vi "柱塞泵调试界面.vi"() -> ()   [LabVIEW 2016, in "质控单元.lvlib"]
uses:
  <vilib>/Utility/miscctls.llb/LVPointTypeDef.ctl
  <vilib>/Analysis/6fits.llb/Curve Fitting Criteria.ctl
  <vilib>/Analysis/NI_AALPro.lvlib
panel:
  out "柱塞泵5体积":dbl
  out "柱塞泵4体积":dbl
  out "柱塞泵3体积":dbl
  out "柱塞泵2体积":dbl
  out "柱塞泵1体积":dbl
  in  "B 5":dbl caption="B5"
  in  "K 5":dbl caption="K5"
  in  "柱塞泵5":bool
  out "关闭 2":bool=TRUE
  in  "枚举":enum16{"柱塞泵1", "柱塞泵2", "柱塞泵3", "柱塞泵4"}(ring)
  in  "柱塞泵4":bool
  in  "柱塞泵3":bool
  in  "柱塞泵2":bool
  in  "柱塞泵1":bool
  out "线性值":T1
  in  "读取":bool
  in  "写入":bool
  in  "柱塞泵枚举":enum16{"柱塞泵1", "柱塞泵2", "柱塞泵3", "柱塞泵4", "柱塞泵5"}(ring)
  in  "启用计算":bool
  in  "标准体积 2":dbl
  in  "标准体积 3":dbl
  in  "实际体积 1":dbl
  in  "实际体积 2":dbl
  in  "实际体积 3":dbl
  in  "标准体积 4":dbl
  in  "实际体积 4":dbl
  in  "标准体积 5":dbl
  in  "实际体积 5":dbl
  in  "标准体积 1":dbl
  out "拟合方程":string
  out "r^2":dbl format="%_6g"
  in  "B 4":dbl caption="B4"
  in  "K 4":dbl caption="K4"
  in  "B 3":dbl caption="B3"
  in  "K 3":dbl caption="K3"
  in  "B 2":dbl caption="B2"
  in  "K 2":dbl caption="K2"
  in  "B":dbl caption="B1"
  in  "K":dbl caption="K1"
  in  "关闭":bool
  # "柱塞泵手动调试计算界面"
  # "柱塞泵启动控制"
  # "柱塞泵体积："
  # "柱塞泵5点线性计算"
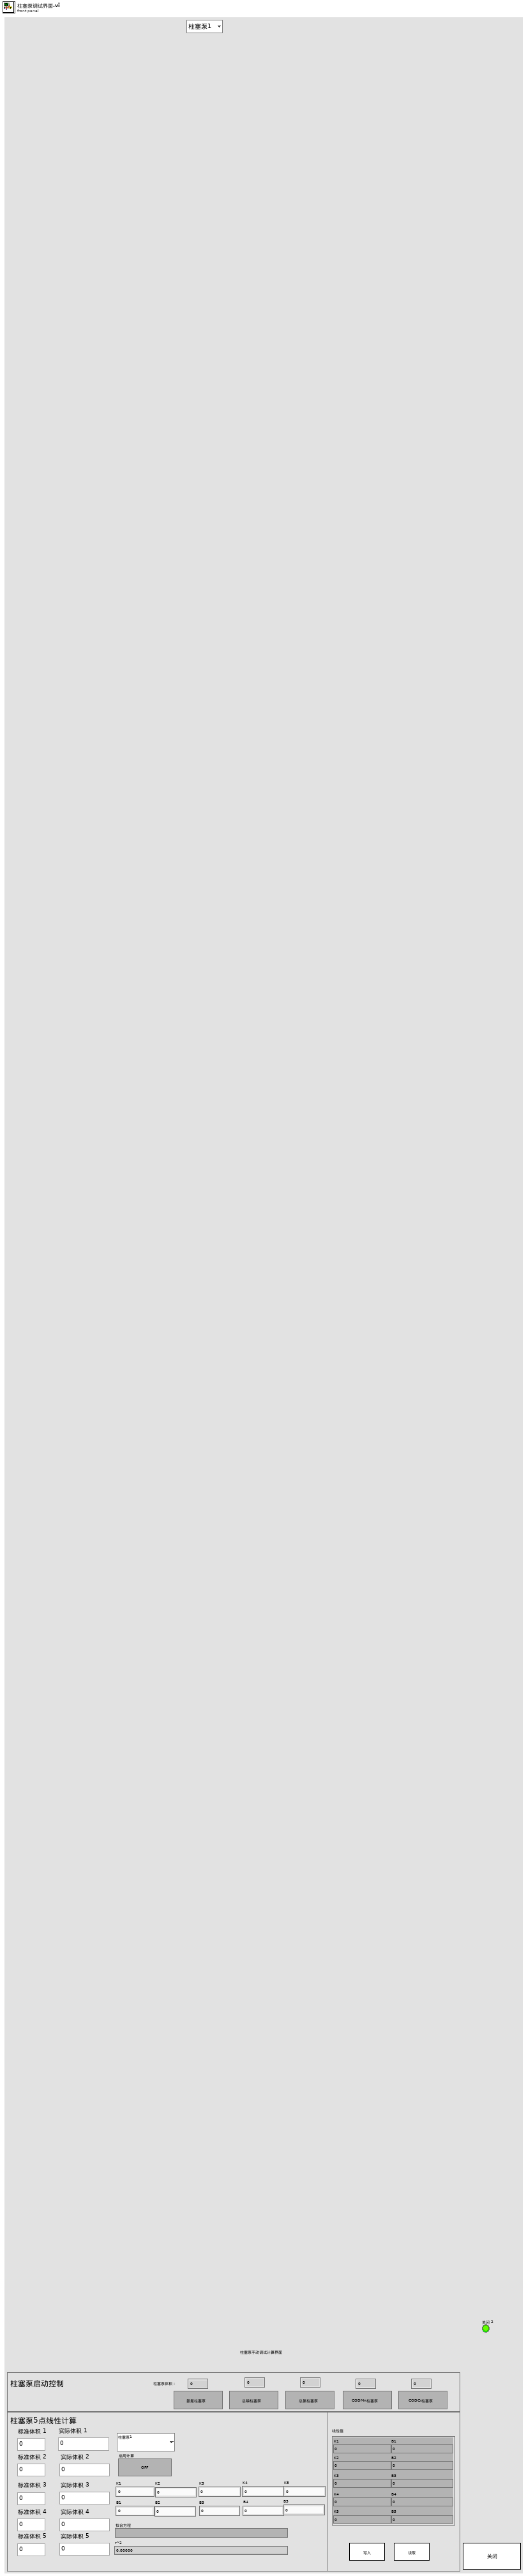
[diagram p1: front panel]
types:
  T1 = cluster{"K1":sgl, "B1":sgl, "K2":sgl, "B2":sgl, "K3":sgl, "B3":sgl, "K4":sgl, "B4":sgl, "K5":sgl, "B5":sgl}
  T2 = typedef "LVPointTypeDef.ctl" = cluster{"Horizontal":i16, "Vertical":i16}
  T3 = typedef "NI_AALPro.lvlib/Curve Fitting Criteria.ctl" = u16
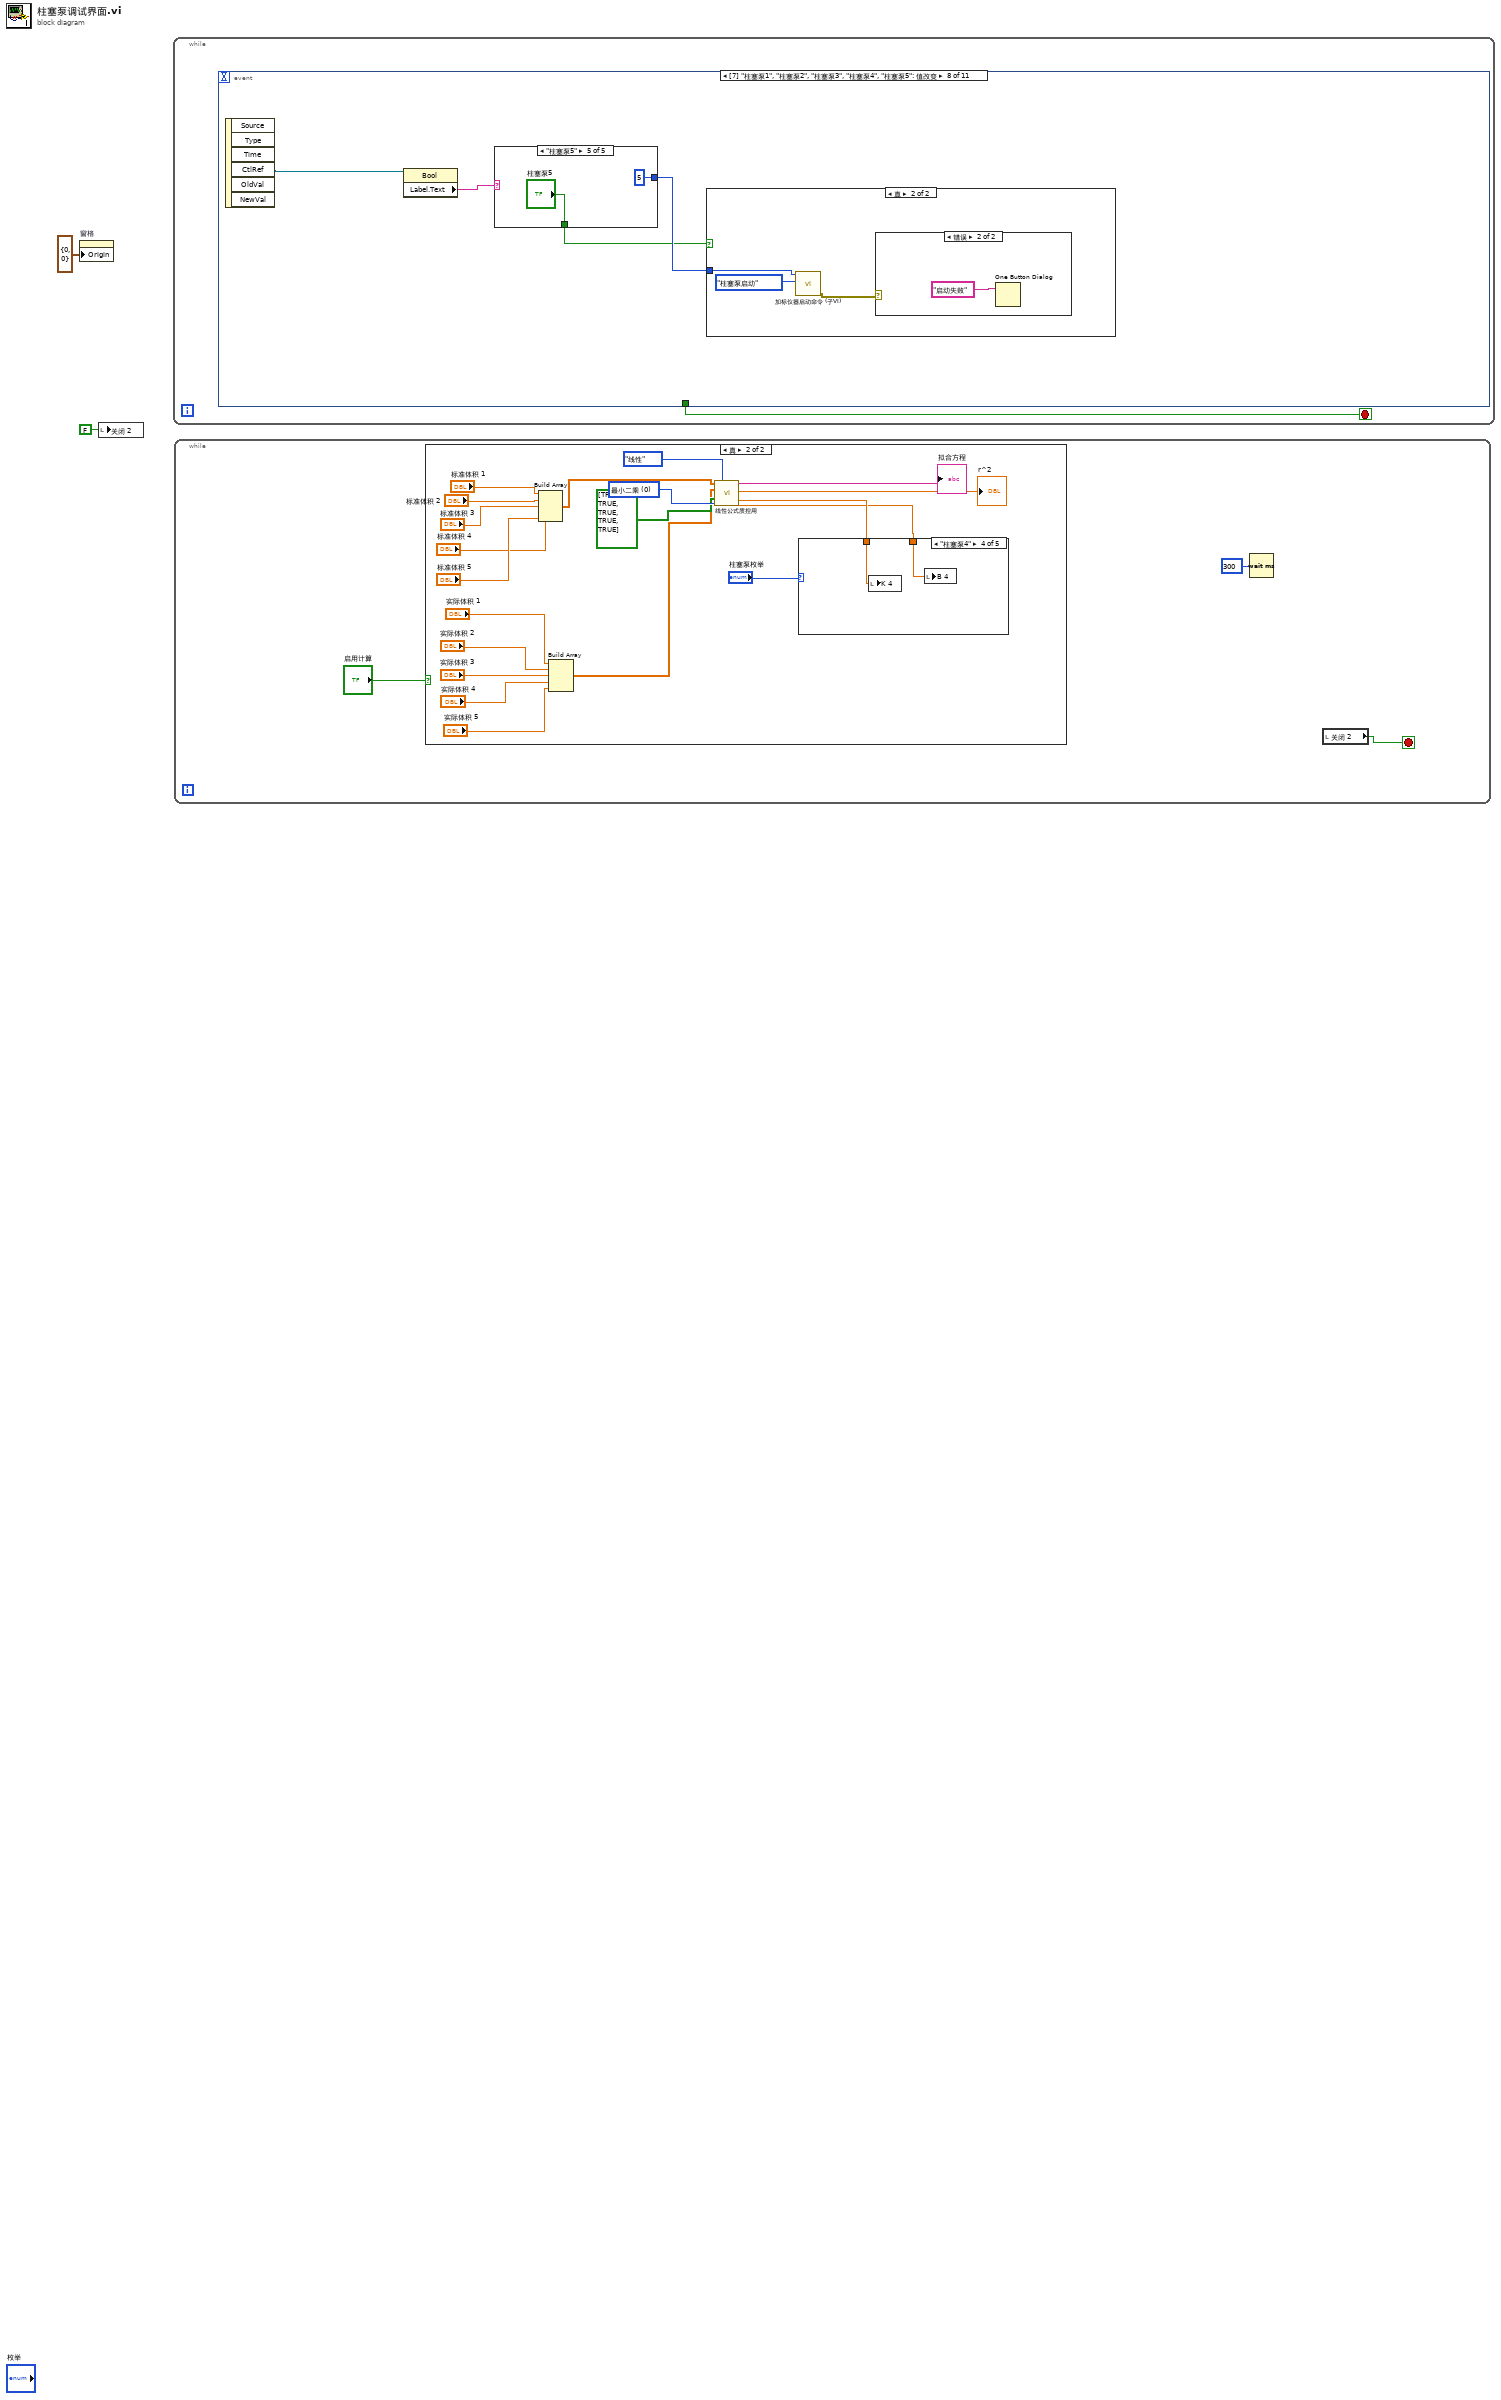
[diagram p0: block diagram]
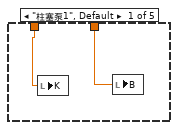
[diagram p3: hidden frame]
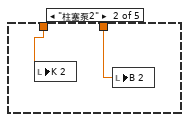
[diagram p4: hidden frame]
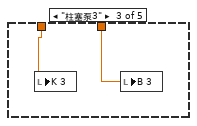
[diagram p5: hidden frame]
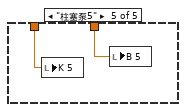
[diagram p6: hidden frame]
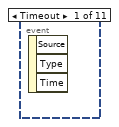
[diagram p7: hidden frame]
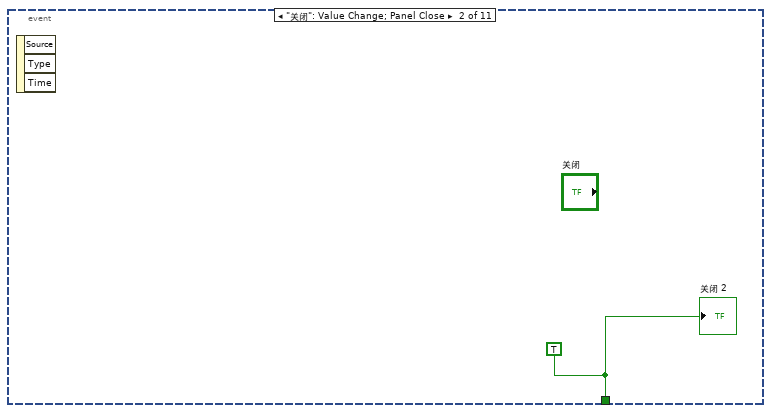
[diagram p8: hidden frame]
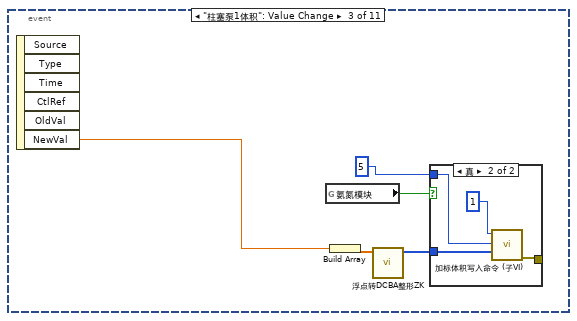
[diagram p9: hidden frame]
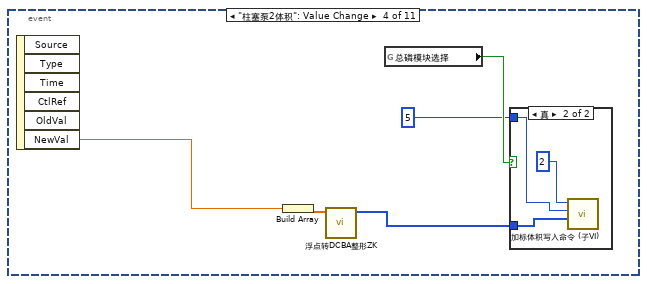
[diagram p11: hidden frame]
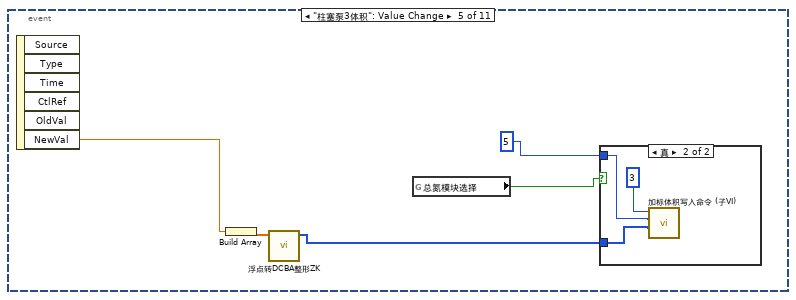
[diagram p13: hidden frame]
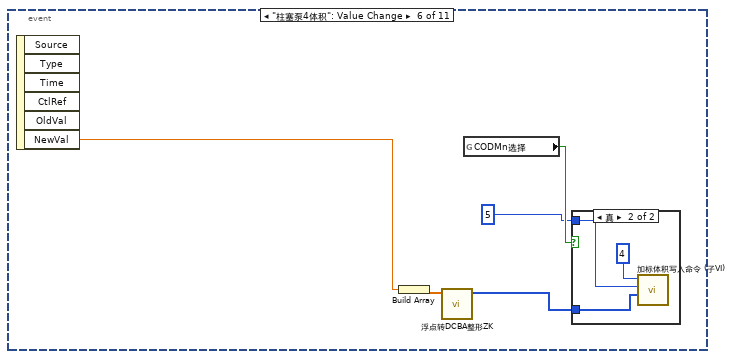
[diagram p15: hidden frame]
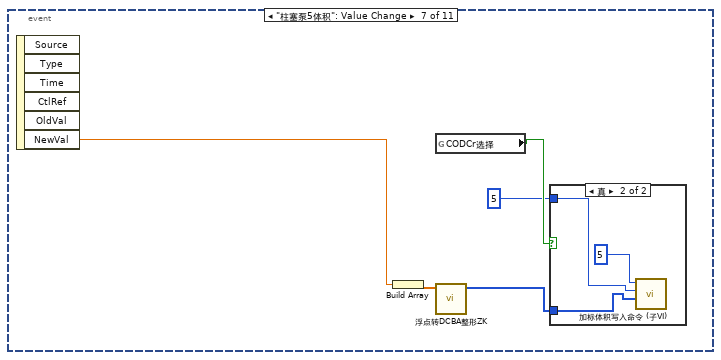
[diagram p17: hidden frame]
diagram:
  n1 = property on="窗格" class="Pane"("Origin"=T2 {"Horizontal"=0, "Vertical"=0} ("原点")) -> ()  [unwired: 2 in, 2 out]
  n2 = local write "关闭 2"(FALSE ("关闭 2")) -> ()
  n3 = while {
    stop <- w3 stop-if-true
    n4 = event shown="[7] \"柱塞泵1\", \"柱塞泵2\", \"柱塞泵3\", \"柱塞泵4\", \"柱塞泵5\": 值改变" {
      selector: _ -> [_ _ _ _ _ _ _ _ _ _ _]
      dyn-events: _ -> [_ _ _ _ _ _ _ _ _ _ _]
      timeout: _ -> [_ _ _ _ _ _ _ _ _ _ _]
      tunnel: [_ w4 _ _ _ _ _ _ _ _ _] -> w3
      event Timeout {
        n5 = event-data() -> ()  [unwired: 1 in, 3 out]
      }
      event "关闭": Value Change; Panel Close {
        w4 = TRUE ("关闭")
        n6 = event-data() -> ()  [unwired: 1 in, 3 out]
        "关闭 2" <- w4
      }
      event "柱塞泵1体积": Value Change {
        n7 = event-data() -> ("NewVal"=w5:dbl)  [unwired: 1 in, 5 out]
        n8 = global read "断电保存全局.vi" "氨氮模块"() -> (w9:bool)
        n9 = Build Array(w5) -> (w8:dbl[])
        n10 = call "浮点转DCBA整形ZK.vi"("浮点数"=w8) -> ("DCBA整形输出"=w7:u16[])  [unwired: 10 in]
        n11 = case shown="真" w9 {
          tunnel: [_ w10] -> _
          tunnel: w7 -> [_ w11]
          tunnel: u16 5 ("starting address") -> [_ w12]
          frame False {
          }
          frame True {
            n12 = call "加标体积写入命令 (子VI).vi"("values"=w11, "starting address"=w12, "Slave ID"=u8 1) -> ("错误输出"=w10:errorcluster)  [unwired: 8 in]
          }
        }
      }
      event "柱塞泵2体积": Value Change {
        n13 = event-data() -> ("NewVal"=w14:dbl)  [unwired: 1 in, 5 out]
        n14 = Build Array(w14) -> (w16:dbl[])
        n15 = call "浮点转DCBA整形ZK.vi"("浮点数"=w16) -> ("DCBA整形输出"=w15:u16[])  [unwired: 10 in]
        n16 = global read "断电保存全局.vi" "总磷模块选择"() -> (w18:bool)
        n17 = case shown="真" w18 {
          tunnel: u16 5 ("starting address") -> [_ w20]
          tunnel: w15 -> [_ w19]
          frame False {
          }
          frame True {
            n18 = call "加标体积写入命令 (子VI).vi"("values"=w19, "starting address"=w20, "Slave ID"=u8 2) -> ()  [unwired: 8 in, 1 out]
          }
        }
      }
      event "柱塞泵3体积": Value Change {
        n19 = event-data() -> ("NewVal"=w22:dbl)  [unwired: 1 in, 5 out]
        n20 = Build Array(w22) -> (w26:dbl[])
        n21 = call "浮点转DCBA整形ZK.vi"("浮点数"=w26) -> ("DCBA整形输出"=w23:u16[])  [unwired: 10 in]
        n22 = global read "断电保存全局.vi" "总氮模块选择"() -> (w24:bool)
        n23 = case shown="真" w24 {
          tunnel: u16 5 ("starting address") -> [_ w28]
          tunnel: w23 -> [_ w27]
          frame False {
          }
          frame True {
            n24 = call "加标体积写入命令 (子VI).vi"("values"=w27, "starting address"=w28, "Slave ID"=u8 3) -> ()  [unwired: 8 in, 1 out]
          }
        }
      }
      event "柱塞泵4体积": Value Change {
        n25 = event-data() -> ("NewVal"=w31:dbl)  [unwired: 1 in, 5 out]
        n26 = Build Array(w31) -> (w32:dbl[])
        n27 = call "浮点转DCBA整形ZK.vi"("浮点数"=w32) -> ("DCBA整形输出"=w30:u16[])  [unwired: 10 in]
        n28 = global read "断电保存全局.vi" "CODMn选择"() -> (w34:bool)
        n29 = case shown="真" w34 {
          tunnel: u16 5 ("starting address") -> [_ w36]
          tunnel: w30 -> [_ w35]
          frame False {
          }
          frame True {
            n30 = call "加标体积写入命令 (子VI).vi"("values"=w35, "starting address"=w36, "Slave ID"=u8 4) -> ()  [unwired: 8 in, 1 out]
          }
        }
      }
      event "柱塞泵5体积": Value Change {
        n31 = event-data() -> ("NewVal"=w40:dbl)  [unwired: 1 in, 5 out]
        n32 = Build Array(w40) -> (w41:dbl[])
        n33 = global read "断电保存全局.vi" "CODCr选择"() -> (w42:bool)
        n34 = call "浮点转DCBA整形ZK.vi"("浮点数"=w41) -> ("DCBA整形输出"=w39:u16[])  [unwired: 10 in]
        n35 = case shown="真" w42 {
          tunnel: u16 5 ("starting address") -> [_ w44]
          tunnel: w39 -> [_ w43]
          frame False {
          }
          frame True {
            n36 = call "加标体积写入命令 (子VI).vi"("values"=w43, "starting address"=w44, "Slave ID"=u8 5) -> ()  [unwired: 8 in, 1 out]
          }
        }
      }
      event "柱塞泵1", "柱塞泵2", "柱塞泵3", "柱塞泵4", "柱塞泵5": Value Change {
        n37 = event-data() -> ("CtlRef"=w48:refnum<vi>)  [unwired: 1 in, 5 out]
        n38 = property class="Bool"(reference=w48) -> ("Label.Text"=w49:string)  [unwired: 1 in, 2 out]
        n39 = case shown="\"柱塞泵5\"" w49 {
          tunnel: [u8 1 ("Slave ID") u8 2 ("Slave ID") u8 3 ("Slave ID") u8 4 ("Slave ID") u8 5 ("Slave ID")] -> w47
          tunnel: ["柱塞泵1" "柱塞泵2" "柱塞泵3" "柱塞泵4" "柱塞泵5"] -> w46
          frame "柱塞泵1", Default {
          }
          frame "柱塞泵2" {
          }
          frame "柱塞泵3" {
          }
          frame "柱塞泵4" {
          }
          frame "柱塞泵5" {
          }
        }
        n40 = case shown="真" w46 {
          tunnel: w47 -> [_ w52]
          frame False {
          }
          frame True {
            n41 = call "加标仪器启动命令 (子VI).vi"("启动命令"=enum16{"启动水样流程", "启动加标流程", "排液", "停止", "柱塞泵启动"}."柱塞泵启动", "仪器"=w52) -> ("错误输出"=w51:errorcluster)  [unwired: 9 in]
            n42 = case shown="错误" w51 {
              frame No Error {
              }
              frame Error {
                n43 = One Button Dialog(message="启动失败" ("消息")) -> ()  [unwired: 1 in, 1 out]
              }
            }
          }
        }
      }
      event "标准体积 1", "实际体积 5", "标准体积 5", "实际体积 4", "标准体积 4", "实际体积 3", "实际体积 2", "实际体积 1", "标准体积 3", "标准体积 2", "线性值.K1", "线性值.B1", "线性值.K2", "线性值.B2", "线性值.K3", "线性值.B3", "线性值.K4", "线性值.B4", "柱塞泵1体积", "柱塞泵2体积", "柱塞泵3体积", "柱塞泵4体积", "柱塞泵5体积": Mouse Down {
        n44 = event-data() -> ("CtlRef"=w67:refnum<vi>)  [unwired: 1 in, 7 out]
        n45 = property class="DigNum"(reference=w67) -> (reference out=w68:refnum<vi>, "Value"=w65:variant)  [unwired: 1 in, 1 out]
        n46 = Variant To Data(type=sgl 0.0 ("NewNumber"), Variant=w65) -> (data=w64:sgl)  [unwired: 1 in, 1 out]
        n47 = call "数字键盘.vi"("OldNumber"=w64) -> ("NewNumber"=w69:sgl)
        n48 = property class="DigNum"(reference=w68, "Val(Sgnl)"=w69) -> ()  [unwired: 1 in, 2 out]
      }
      event "写入": Value Change {
        n49 = event-data() -> ()  [unwired: 1 in, 6 out]
        n50 = control-ref of="柱塞泵枚举"() -> (w73:refnum<vi>)
        n51 = property class="Enum (严格)"(reference=w73) -> ("RingText.Text"=w72:string)  [unwired: 1 in, 2 out]
        n52 = Concatenate Strings("是否将K、B值写入" ("字符串"), w72, "？" ("字符串")) -> (w70:string)
        n53 = Two Button Dialog(message=w70) -> (T button?=w75:bool)  [unwired: 2 in]
        n54 = case shown="真" w75 {
          frame False {
          }
          frame True {
            n55 = local read "柱塞泵枚举"() -> (w76:enum16{"柱塞泵1", "柱塞泵2", "柱塞泵3", "柱塞泵4", "柱塞泵5"})
            n56 = case shown="\"柱塞泵1\", 默认" w76 {
              tunnel: [w82 w90 w97 w104 w110] -> w77
              frame "柱塞泵1", Default {
                n57 = Build Array("K", "B") -> (w79:dbl[])
                n58 = call "浮点转DCBA整形ZK.vi"("浮点数"=w79) -> ("DCBA整形输出"=w78:u16[])  [unwired: 10 in]
                n59 = call "写入参数.vi"("values"=w78, "starting address"=u16 1, "Slave ID"=u8 1) -> ("error out"=w82:errorcluster)  [unwired: 8 in]
              }
              frame "柱塞泵2" {
                n60 = Build Array("K 2", "B 2") -> (w86:dbl[])
                n61 = call "浮点转DCBA整形ZK.vi"("浮点数"=w86) -> ("DCBA整形输出"=w85:u16[])  [unwired: 10 in]
                n62 = call "写入参数.vi"("values"=w85, "starting address"=u16 1, "Slave ID"=u8 2) -> ("error out"=w90:errorcluster)  [unwired: 8 in]
              }
              frame "柱塞泵3" {
                n63 = Build Array("K 3", "B 3") -> (w93:dbl[])
                n64 = call "浮点转DCBA整形ZK.vi"("浮点数"=w93) -> ("DCBA整形输出"=w92:u16[])  [unwired: 10 in]
                n65 = call "写入参数.vi"("values"=w92, "starting address"=u16 1, "Slave ID"=u8 3) -> ("error out"=w97:errorcluster)  [unwired: 8 in]
              }
              frame "柱塞泵4" {
                n66 = Build Array("K 4", "B 4") -> (w100:dbl[])
                n67 = call "浮点转DCBA整形ZK.vi"("浮点数"=w100) -> ("DCBA整形输出"=w99:u16[])  [unwired: 10 in]
                n68 = call "写入参数.vi"("values"=w99, "starting address"=u16 1, "Slave ID"=u8 4) -> ("error out"=w104:errorcluster)  [unwired: 8 in]
              }
              frame "柱塞泵5" {
                n69 = Build Array("K 5", "B 5") -> (w107:dbl[])
                n70 = call "浮点转DCBA整形ZK.vi"("浮点数"=w107) -> ("DCBA整形输出"=w106:u16[])  [unwired: 10 in]
                n71 = call "写入参数.vi"("values"=w106, "starting address"=u16 1, "Slave ID"=u8 5) -> ("error out"=w110:errorcluster)  [unwired: 8 in]
              }
            }
            n72 = case shown="无错误" w77 {
              frame No Error {
                n73 = One Button Dialog(message="写入成功" ("消息"), button name ("OK")="确定" ("按钮名称（“确定”）")) -> ()  [unwired: 1 out]
              }
              frame Error {
                n74 = One Button Dialog(message="写入失败" ("消息"), button name ("OK")="确定" ("按钮名称（“确定”）")) -> ()  [unwired: 1 out]
              }
            }
          }
        }
      }
      event "读取": Value Change {
        n75 = event-data() -> ()  [unwired: 1 in, 6 out]
        n76 = local read "线性值"() -> (w117:T1)
        n77 = global read "断电保存全局.vi" "氨氮模块"() -> (w138:bool)
        n78 = case shown="真" w138 {
          tunnel: [errorcluster {"status"=FALSE, "code"=0, "source"=""} ("error out") w176] -> w129
          tunnel: [w169 w175] -> w130
          tunnel: [w168 w174] -> w131
          tunnel: w117 -> [w167 _]
          frame False {
            n79 = Unbundle By Name(w167) -> ("K1"=w169:sgl, "B1"=w168:sgl)
          }
          frame True {
            n80 = call "读取参数.vi"("Slave ID"=u8 1, "starting address"=u16 1, "quantity"=u16 6) -> ("values"=w173:u16[], "error out"=w176:errorcluster)  [unwired: 6 in]
            n81 = call "HexToDCBAFloat.vi"("数组"=w173) -> ("FLOAT"=w172:sgl[])  [unwired: 10 in]
            n82 = Index Array(array=w172) -> (element #1=w175:sgl, element #2=w174:sgl, element #3=→"柱塞泵1体积":sgl)  [unwired: 3 in]
          }
        }
        n83 = global read "断电保存全局.vi" "总磷模块选择"() -> (w128:bool)
        n84 = case shown="真" w128 {
          tunnel: w129 -> [w181 w192]
          tunnel: [w181 w191] -> w122
          tunnel: [w183 w190] -> w132
          tunnel: [w182 w189] -> w133
          tunnel: w117 -> [w180 _]
          frame False {
            n85 = Unbundle By Name(w180) -> ("K2"=w183:sgl, "B2"=w182:sgl)
          }
          frame True {
            n86 = call "读取参数.vi"("Slave ID"=u8 2, "starting address"=u16 1, "quantity"=u16 6, "Error in"=w192) -> ("values"=w186:u16[], "error out"=w191:errorcluster)  [unwired: 5 in]
            n87 = call "HexToDCBAFloat.vi"("数组"=w186) -> ("FLOAT"=w185:sgl[])  [unwired: 10 in]
            n88 = Index Array(array=w185) -> (element #1=w190:sgl, element #2=w189:sgl, element #3=→"柱塞泵2体积":sgl)  [unwired: 3 in]
          }
        }
        n89 = global read "断电保存全局.vi" "总氮模块选择"() -> (w121:bool)
        n90 = case shown="真" w121 {
          tunnel: w122 -> [w140 w151]
          tunnel: [w140 w150] -> w120
          tunnel: [w142 w149] -> w119
          tunnel: [w141 w148] -> w118
          tunnel: w117 -> [w139 _]
          frame False {
            n91 = Unbundle By Name(w139) -> ("K3"=w142:sgl, "B3"=w141:sgl)
          }
          frame True {
            n92 = call "读取参数.vi"("Slave ID"=u8 3, "starting address"=u16 1, "quantity"=u16 6, "Error in"=w151) -> ("values"=w145:u16[], "error out"=w150:errorcluster)  [unwired: 5 in]
            n93 = call "HexToDCBAFloat.vi"("数组"=w145) -> ("FLOAT"=w144:sgl[])  [unwired: 10 in]
            n94 = Index Array(array=w144) -> (element #1=w149:sgl, element #2=w148:sgl, element #3=→"柱塞泵3体积":sgl)  [unwired: 3 in]
          }
        }
        n95 = global read "断电保存全局.vi" "CODMn选择"() -> (w137:bool)
        n96 = case shown="真" w137 {
          tunnel: w120 -> [w195 w206]
          tunnel: [w197 w205] -> w124
          tunnel: [w196 w204] -> w123
          tunnel: [w195 w201] -> w134
          tunnel: w117 -> [w194 _]
          frame False {
            n97 = Unbundle By Name(w194) -> ("K4"=w197:sgl, "B4"=w196:sgl)
          }
          frame True {
            n98 = call "读取参数.vi"("Slave ID"=u8 4, "starting address"=u16 1, "quantity"=u16 6, "Error in"=w206) -> ("values"=w200:u16[], "error out"=w201:errorcluster)  [unwired: 5 in]
            n99 = call "HexToDCBAFloat.vi"("数组"=w200) -> ("FLOAT"=w199:sgl[])  [unwired: 10 in]
            n100 = Index Array(array=w199) -> (element #1=w205:sgl, element #2=w204:sgl, element #3=→"柱塞泵4体积":sgl)  [unwired: 3 in]
          }
        }
        n101 = global read "断电保存全局.vi" "CODCr选择"() -> (w136:bool)
        n102 = case shown="真" w136 {
          tunnel: w134 -> [w154 w165]
          tunnel: [w156 w164] -> w126
          tunnel: [w155 w163] -> w125
          tunnel: [w154 w160] -> w135
          tunnel: w117 -> [w153 _]
          frame False {
            n103 = Unbundle By Name(w153) -> ("K5"=w156:sgl, "B5"=w155:sgl)
          }
          frame True {
            n104 = call "读取参数.vi"("Slave ID"=u8 5, "starting address"=u16 1, "quantity"=u16 6, "Error in"=w165) -> ("values"=w159:u16[], "error out"=w160:errorcluster)  [unwired: 5 in]
            n105 = call "HexToDCBAFloat.vi"("数组"=w159) -> ("FLOAT"=w158:sgl[])  [unwired: 10 in]
            n106 = Index Array(array=w158) -> (element #1=w164:sgl, element #2=w163:sgl, element #3=→"柱塞泵5体积":sgl)  [unwired: 3 in]
          }
        }
        n107 = Bundle By Name(cluster=w117, "K1"=w130, "B1"=w131, "K2"=w132, "B2"=w133, "K3"=w119, "B3"=w118, "K4"=w124, "B4"=w123, "K5"=w126, "B5"=w125) -> (→"线性值":T1)
        n108 = case shown="无错误" w135 {
          frame No Error {
            n109 = One Button Dialog(message="读取成功" ("消息"), button name ("OK")="确定" ("按钮名称（“确定”）")) -> ()  [unwired: 1 out]
          }
          frame Error {
            n110 = One Button Dialog(message="读取失败" ("消息"), button name ("OK")="确定" ("按钮名称（“确定”）")) -> ()  [unwired: 1 out]
          }
        }
      }
    }
  }
  n111 = while {
    stop <- w213 stop-if-true
    n112 = case shown="真" "启用计算" {
      frame False {
      }
      frame True {
        w231 = T3 0 items=["最小二乘", "最小绝对残差", "Bisquare"] ("method")
        n113 = Build Array("标准体积 1", "标准体积 2", "标准体积 3", "标准体积 4", "标准体积 5") -> (w228:dbl[])
        n114 = Build Array("实际体积 1", "实际体积 2", "实际体积 3", "实际体积 4", "实际体积 5") -> (w229:dbl[])
        n115 = call "线性公式质控用.vi"("标液浓度"=w228, "模型"=enum32{"线性", "多项式"}."线性", "监测浓度"=w229, "启用"=bool[] [TRUE, TRUE, TRUE, TRUE, TRUE], "method"=w231) -> ("拟合方程"=→"拟合方程":string, "r^2"=→"r^2":dbl, "slope"=w217:dbl, "intercept"=w216:dbl)  [unwired: 6 in, 1 out]
        n116 = case shown="\"柱塞泵4\"" "柱塞泵枚举" {
          tunnel: w217 -> [w235 w238 w239 w242 w244]
          tunnel: w216 -> [w236 w237 w240 w241 w243]
          frame "柱塞泵1", Default {
            n117 = local write "K"(w235) -> ()
            n118 = local write "B"(w236) -> ()
          }
          frame "柱塞泵2" {
            n119 = local write "K 2"(w238) -> ()
            n120 = local write "B 2"(w237) -> ()
          }
          frame "柱塞泵3" {
            n121 = local write "K 3"(w239) -> ()
            n122 = local write "B 3"(w240) -> ()
          }
          frame "柱塞泵4" {
            n123 = local write "K 4"(w242) -> ()
            n124 = local write "B 4"(w241) -> ()
          }
          frame "柱塞泵5" {
            n125 = local write "K 5"(w244) -> ()
            n126 = local write "B 5"(w243) -> ()
          }
        }
      }
    }
    n127 = Wait (ms)(milliseconds to wait=u32 300 ("等待时间（毫秒）")) -> ()  [unwired: 1 out]
    n128 = local read "关闭 2"() -> (w213:bool)
  }
